vi "PWMTest.vi"() -> ()   [LabVIEW 2009]
uses:
  <vilib>/rvi/interface/nirviOpenFPGA/nirviOpenFPGA.xnode
  FPGA Bitfiles/scmproject.lvproj_FPGA Target_RobotFPGA.vi.lvbitx
  RobotFPGA.vi
  <vilib>/FPGAPlugInAG/cRIO-9074/nirviIntfOpen_cRIO-9074.vi
  <vilib>/Platform/TimedLoop/XDataNode/XDataNode.xnode
  <vilib>/Platform/TimedLoop/XDataNode/loadlvalarms.vi
  <vilib>/Platform/TimedLoop/XDataNode/timing_clust.ctl
  <vilib>/Platform/TimedLoop/XDataNode/nitl_modes.ctl
  <vilib>/Platform/TimedLoop/XDataNode/wakeup.ctl
  <vilib>/rvi/interface/nirviReadWriteControl/nirviReadWriteControl.xnode
  <vilib>/LabVIEW Targets/FPGA/Rio/nirio_HostInterface/nirio_WriteBig.vi
  <vilib>/Utility/error.llb/Error Cluster From Error Code.vi
  <vilib>/rvi/errors/niLvFpgaAdjustHostInterfaceError.vi
  <vilib>/rvi/interface/common/niFpgaNodeNameForErrorReporting.ctl
  <vilib>/rvi/errors/niLvFpgaWhatHappensToTopLevelVI.ctl
  <vilib>/rvi/interface/nirviCloseFPGA/nirviCloseFPGA.xnode
  <vilib>/FPGAPlugInAG/cRIO-9074/nirviIntfClose_cRIO-9074.vi
  <vilib>/Platform/TimedLoop/XDataNode/XDNodeRunTimeDep.lvlib
  <vilib>/userdefined/High Color/nirio_resource_hc.ctl
  NiRioSrv.dll
panel:
  in  "PWM1_Enable":bool
  in  "PWM1":cluster{"High (uSec)":u32, "Period (uSec)":u32} {"High (uSec)" scale=900.0..2100.0}
  in  "PWM10_Enable":bool
  in  "PWM9_Enable":bool
  in  "PWM10":cluster{"High (uSec)":u32, "Period (uSec)":u32}={"High (uSec)"=1360, "Period (uSec)"=0} {"High (uSec)" min=1360 max=2200 scale=1360.0..2200.0}
  in  "PWM9":cluster{"High (uSec)":u32, "Period (uSec)":u32}={"High (uSec)"=930, "Period (uSec)"=0} {"High (uSec)" min=930 max=1770 scale=930.0..1770.0}
  in  "stop":bool
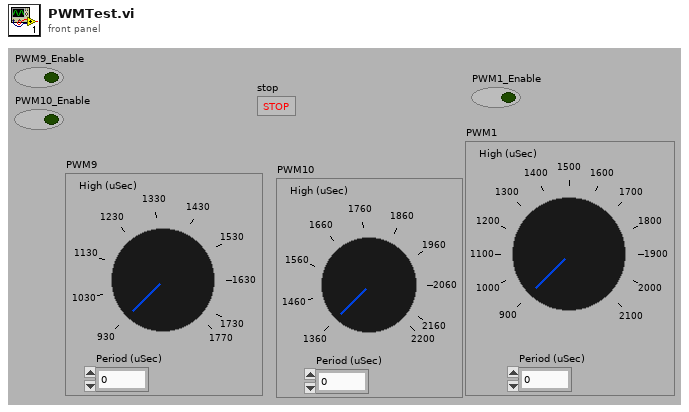
[diagram p1: front panel]
types:
  T1 = cluster{"signature":u8[], "vi signatures match":bool, "signature register address":u32, "reset register address":u32, "control register address":u32, "interrupt base address":u32, "Bitstream Version":u32, "DMA Configuration":cluster{"Name":string, "Depth":u32, "Write? (Deprecated:Use Implementation)":bool, "Physical Channel":u32, "Base Address":u32, "Data Width":u32, "Data Type":enum32{"Boolean", "I8", "I16", "I32", "I64", "U8", "U16", "U32", "U64", "FXP"}, "FXP Properties":variant, "Write Window Address":u32, "Implementation":enum16{"niFpgaTargetToHost", "niFpgaHostToTarget", "niFpgaPeerToPeerWriter", "niFpgaPeerToPeerReader", "niCoreTargetToHost", "niCoreHostToTarget"}, "Control Set":u32}[], "run when loaded?":bool, "reset register size in bits":u32, "compilation results xml":string}
  T2 = typedef "niFpgaNodeNameForErrorReporting.ctl" = enum16{"Open FPGA VI Reference", "Read/Write Control", "Invoke Method: Abort", "Invoke Method: Acknowledge IRQ", "Invoke Method: Download", "Invoke Method: FIFO.Configure", "Invoke Method: FIFO.Read", "Invoke Method: FIFO.Start", "Invoke Method: FIFO.Stop", "Invoke Method: FIFO.Write", "Invoke Method: Reset", "Invoke Method: Run", "Invoke Method: Wait on IRQ", "Close FPGA VI Reference"}
  T3 = typedef "niLvFpgaWhatHappensToTopLevelVI.ctl" = enum16{"top level VI scripted behind XNode", "top level VI inlined behind XNode"}
  T4 = typedef "XDNodeRunTimeDep.lvlib/timing_clust.ctl" = cluster{"Expected End [f-1]":u64, "Actual End [f-1]":u64, "Finished Late? [f-1]":bool, "Expected End [i-1]":u64, "Actual End [i-1]":u64, "Finished Late? [i-1]":bool, "Expected Start [i]":u64, "Actual Start [i]":u64, "Expected Start [f]":u64, "Actual Start [f]":u64, "Source Name":string, "Structure Name":string, "Period":i64, "Deadline":i64, "Offset":i64, "Start":i64, "Priority":i32, "Timeout":i32, "Mode":T5, "Wakeup Reason":T6, "Error":errorcluster, "Source Type":string, "Secondary Source Type":string, "Global End Time":u64, "Global Start Time":u64, "Frame Duration":u64, "Iteration Duration":u64, "Assigned CPU":i32, "I/O Scan Engine Mode":u32}
  T5 = typedef "XDNodeRunTimeDep.lvlib/nitl_modes.ctl" = enum32{"No Change", "Process missed periods, maintain original phase", "Discard missed periods, maintain original phase", "Process missed periods, ignore original phase", "Discard missed periods, ignore original phase"}
  T6 = typedef "XDNodeRunTimeDep.lvlib/wakeup.ctl" = enum32{"Normal", "Aborted", "Asynchronous wakeup", "Timing source error", "Timed loop error", "Timeout"}
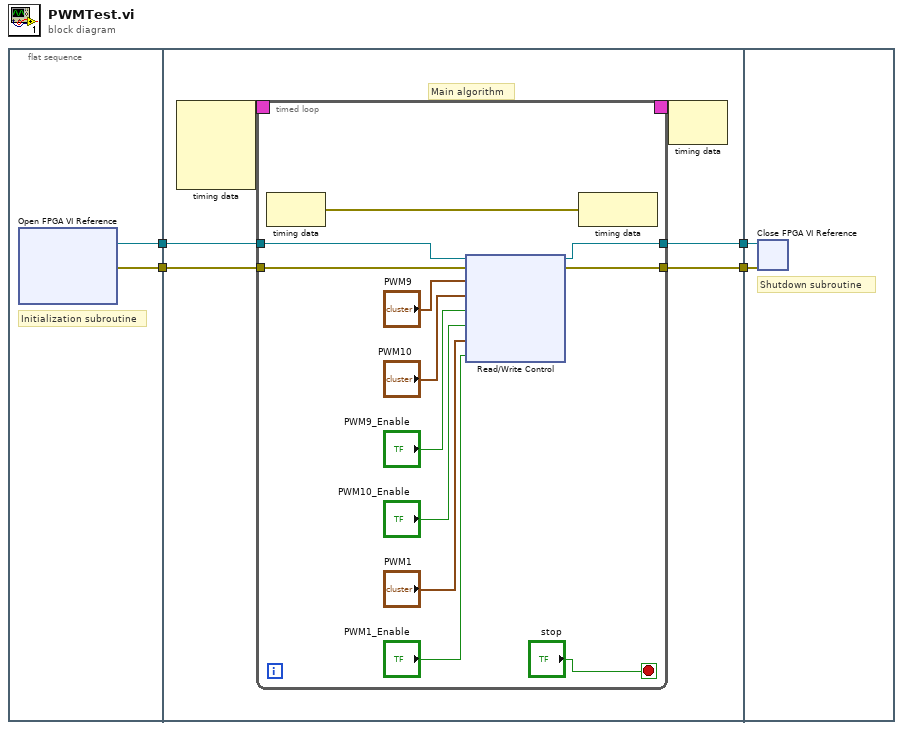
[diagram p0: block diagram]
diagram:
  n1 = flat-sequence {
    tunnel: [w6] -> w4
    tunnel: [w5] -> w3
    tunnel: w4 -> [w21]
    tunnel: w3 -> [w20]
    tunnel: [w19] -> w2
    tunnel: [w18] -> w1
    tunnel: w2 -> [w151]
    tunnel: w1 -> [w150]
    frame #0 {
      # "Initialization subroutine"
      n2 = xnode "Open FPGA VI Reference"() -> ("FPGA VI Reference Out"=w6:refnum<k20>, "error out"=w5:errorcluster)  [unwired: 2 in]
    }
    frame #1 {
      # "Main algorithm"
      n3 = node-c288() -> (w23:T4)  [unwired: 4 in]
      n4 = timed-loop {
        timing: w23 -> [_]
        timing-out: [_] -> w22
        tunnel: w21 -> [w30]
        tunnel: w20 -> [w33]
        tunnel: [w32] -> w19
        tunnel: [w31] -> w18
        stop <- "stop" stop-if-true
        n5 = node-c288() -> (w34:errorcluster)  [unwired: 1 in]
        n6 = xnode "Read/Write Control"("FPGA VI Reference In"=w30, "error in"=w33, "PWM9"="PWM9", "PWM10"="PWM10", "PWM9_Enable"="PWM9_Enable", "PWM10_Enable"="PWM10_Enable", "PWM1"="PWM1", "PWM1_Enable"="PWM1_Enable") -> ("FPGA VI Reference Out"=w32:refnum<k20>, "error out"=w31:errorcluster)
        n7 = node-c288(w34) -> ()  [unwired: 1 out]
      }
      n8 = node-c288(w22) -> ()  [unwired: 1 out]
    }
    frame #2 {
      # "Shutdown subroutine"
      n9 = xnode "Close FPGA VI Reference"("FPGA VI Reference In"=w151, "error in"=w150) -> ()  [unwired: 1 out]
    }
  }
